vi "Cabin.vi"(7 "LVWSR":refnum<class "Web Request.lvclass">, 11 "val":u8) -> ()   [LabVIEW 2014]
uses:
  <vilib>/wsapi/Web Request.lvclass
  Controller/Messages/Change Inlet MSG/Change Inlet MSG.lvclass
  Controller/Messages/Update Switch State MSG/Update Switch MSG.lvclass/Update Switch MSG.ctl
  Controller/Messages/Update Switch State MSG/Write SwitchState.vi
  Controller/Controller.lvclass
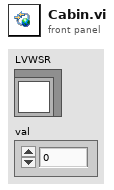
[diagram p1: front panel]
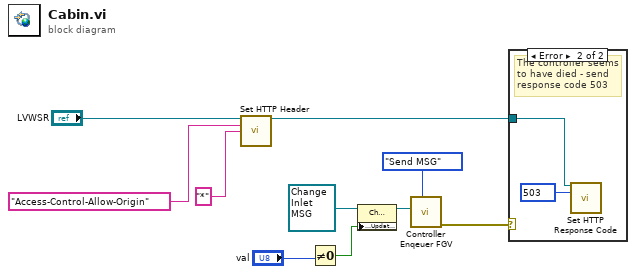
[diagram p0: block diagram]
diagram:
  n1 = call <vilib>:"Set HTTP Header.vi"("LabVIEW Web Service Request"="LVWSR", "header"="Access-Control-Allow-Origin", "header value"="*") -> ("LabVIEW Web Service Request out"=w8:refnum<class "Web Request.lvclass">)  [unwired: 11 in, 1 out]
  n2 = Not Equal To 0?(x="val") -> (x != 0?=w1:bool)
  n3 = property class="Change Inlet MSG.lvclass"(reference=refnum<class "Change Inlet MSG.lvclass"> refnum ("Controller.lvlib:Change Inlet MSG.lvclass"), "Accessors:UpdateSw"=w1) -> (reference out=w3:refnum<class "Change Inlet MSG.lvclass">)  [unwired: 1 in, 1 out]
  n4 = call "Controller Enqeuer FGV.vi"("State"=enum16{"Store", "Send MSG"}."Send MSG", "MSG"=w3) -> ("error out"=w7:errorcluster)  [unwired: 9 in]
  n5 = case shown="Error" w7 {
    tunnel: w8 -> [_ w11]
    frame No Error {
    }
    frame Error {
      w12 = 503 items=["100"=100, "101"=101, "200"=200, "201"=201, "202"=202, "203"=203, "204"=204, "205"=205, "206"=206, "300"=300, "301"=301, "302"=302, "303"=303, "304"=304, "305"=305, "306"=306, "307"=307, "400"=400, "401"=401, "402"=402, "403"=403, "404"=404, "405"=405, "406"=406, "407"=407, "408"=408, "409"=409, "410"=410, "411"=411, "412"=412, "413"=413, "414"=414, "415"=415, "416"=416, "417"=417, "500"=500, "501"=501, "502"=502, "503"=503, "504"=504, "505"=505] ("response code (200)")
      # "The controller seems to have died - send response code 503"
      n6 = call <vilib>:"Set HTTP Response Code.vi"("LabVIEW Web Service Request"=w11, "response code (200)"=w12) -> ()  [unwired: 12 in, 2 out]
    }
  }
